vi "ReadTestList.vi"(10 "Model":string="7534-FE-FCT2") -> (1 "TestList":T1[](array[typedef]), 2 "size(s)":i32)   [LabVIEW 2013]
uses:
  TestVI/TestItemBox.ctl
  TestVI/TestItem.ctl
  Control/Buffer.vi
panel:
  out "Describe":string[](array[string])
  out "TestItem":string[](array[string])
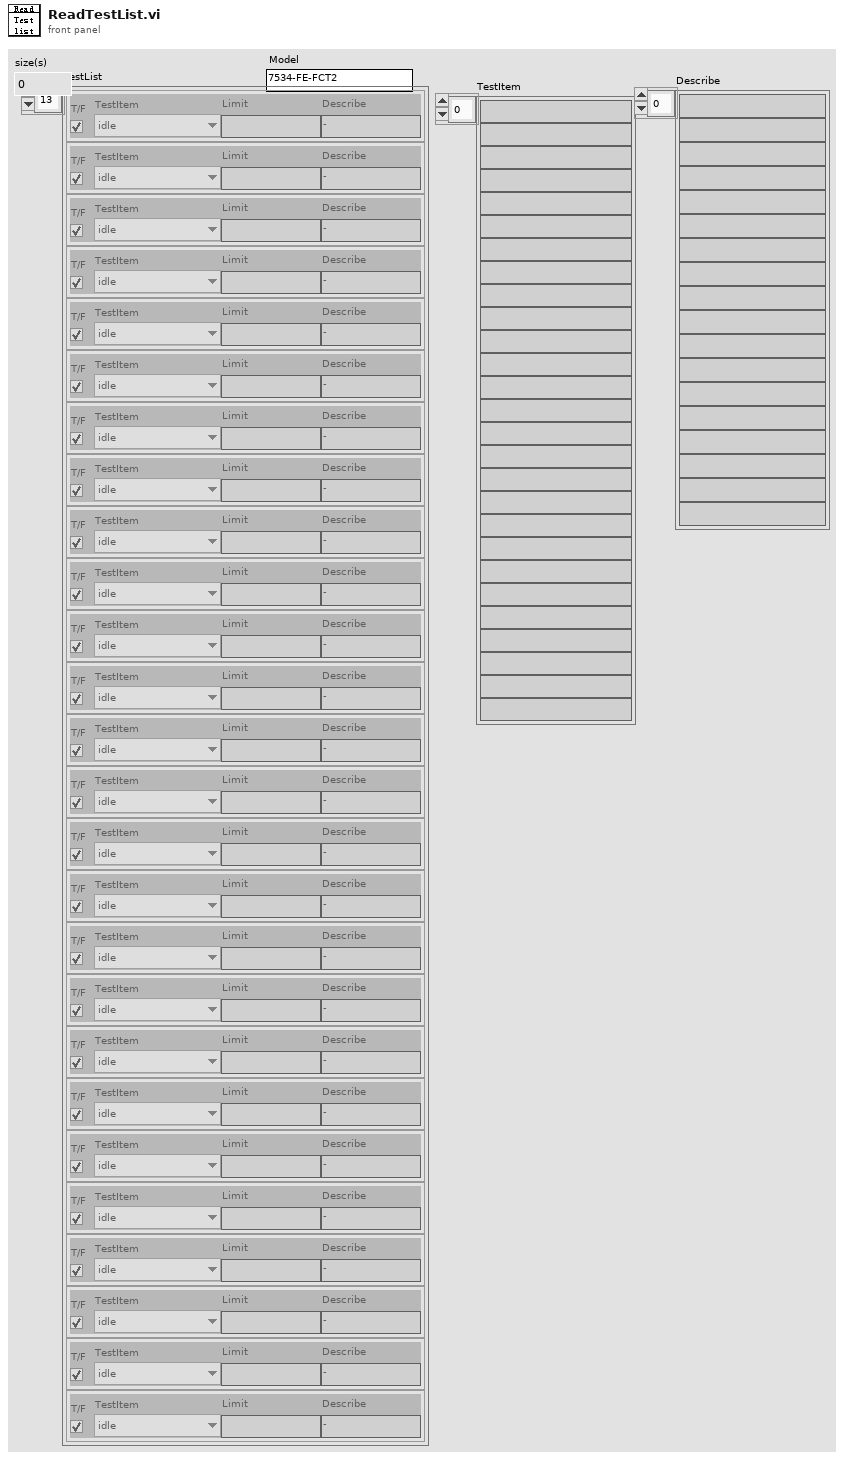
[diagram p1: front panel]
types:
  T1 = typedef "TestItemBox.ctl" = cluster{"T/F":bool, "TestItem":T2, "Limit":string, "Describe":string}
  T2 = typedef "TestItem.ctl" = enum16{"Dynamic_call", "idle", "Dialog", "Check_SF", "Delay", "Reset_HiPot", "HV_Test", "GB_Test", "Instrument_Write&Read_HIPOT", "Hipot_ReadResult", "Hipot_Close", "CheckModel", "ScanTestStart", "ScanMultChannel_DCV", "ScanOneChannel_DCV", "Diplay_TestList"}
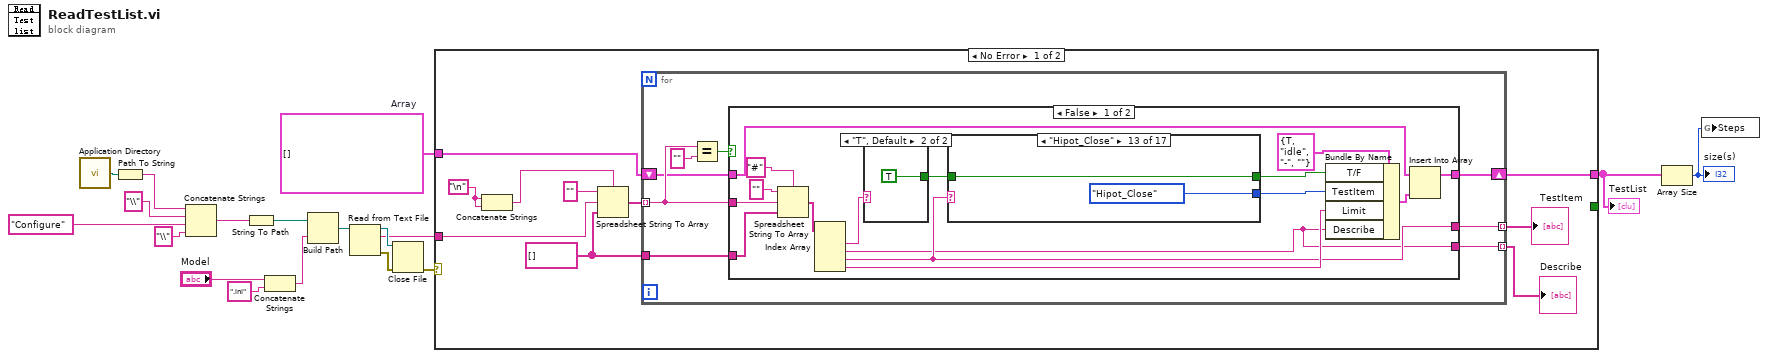
[diagram p0: block diagram]
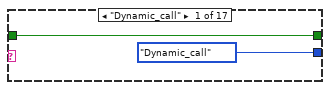
[diagram p2: hidden frame]
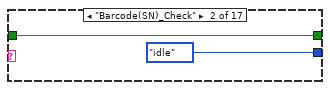
[diagram p3: hidden frame]
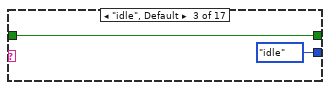
[diagram p4: hidden frame]
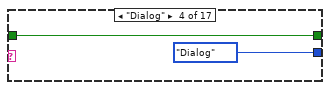
[diagram p5: hidden frame]
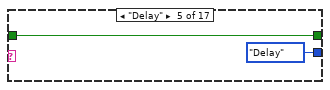
[diagram p6: hidden frame]
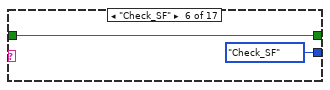
[diagram p7: hidden frame]
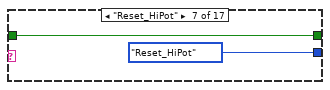
[diagram p8: hidden frame]
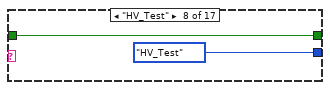
[diagram p9: hidden frame]
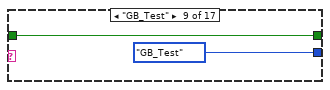
[diagram p10: hidden frame]
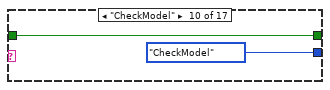
[diagram p11: hidden frame]
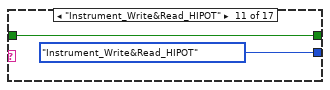
[diagram p12: hidden frame]
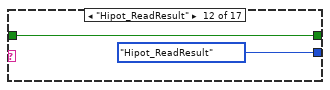
[diagram p13: hidden frame]
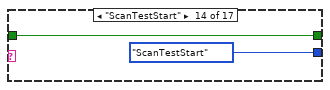
[diagram p14: hidden frame]
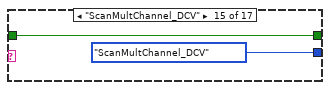
[diagram p15: hidden frame]
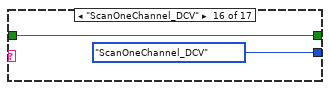
[diagram p16: hidden frame]
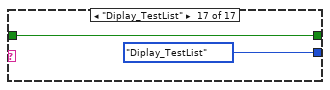
[diagram p17: hidden frame]
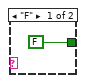
[diagram p18: hidden frame]
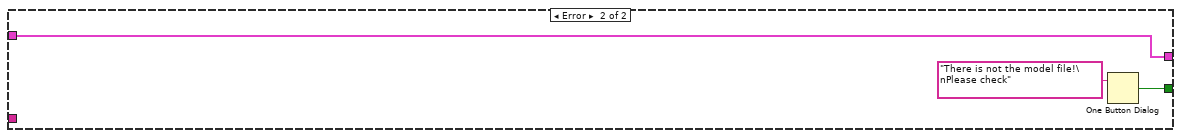
[diagram p20: hidden frame]
diagram:
  w2 = T1[] []  # Array
  n1 = call <vilib>:"Application Directory.vi"() -> ("Application Directory"=w15:path)
  n2 = Path To String(path=w15) -> (string=w14:string)
  n3 = Concatenate Strings(w14, "\\" ("string"), "Configure" ("string"), "\\" ("string")) -> (w11:string)
  n4 = String To Path(string=w11) -> (path=w10:path)
  n5 = Concatenate Strings("Model", ".ini" ("string")) -> (w7:string)
  n6 = Build Path(base path=w10, name or relative path=w7) -> (appended path=w1:path)
  n7 = Read from Text File(file (use dialog)=w1) -> (refnum out=w6:refnum<file>, text=w3:string, error out=w5:errorcluster)  [unwired: 3 in, 1 out]
  n8 = Close File(refnum=w6, error in=w5) -> (error out=w4:errorcluster)  [unwired: 1 out]
  n9 = case shown="No Error" w4 {
    tunnel: w3 -> [w28 _]
    tunnel: w2 -> [w24 w92]
    tunnel: [w23 w92] -> w17
    tunnel: [_ w90] -> _
    frame No Error {
      w22 = "\n"
      w25 = string[] []
      n10 = Concatenate Strings(w22, w22) -> (w21:string)
      n11 = Spreadsheet String To Array(delimiter (Tab)=w21, format string="", spreadsheet string=w28, array type (2D Dbl)=w25) -> (array=w26:string[])
      n12 = for {
        tunnel: w26 -> [w34] mode=indexing
        tunnel: w25 -> [w33]
        shift-right: [w31] -> w23
        shift-left: w24 -> [w32]
        tunnel: [w30] -> w20 mode=indexing
        tunnel: [w29] -> w19 mode=indexing
        n13 = Equal?(x=w34, y="") -> (x = y?=w35:bool)
        n14 = case shown="False" w35 {
          tunnel: w34 -> [w50 _]
          tunnel: w33 -> [w49 _]
          tunnel: w32 -> [w47 w89]
          tunnel: [w45 w89] -> w31
          tunnel: [w38 _] -> w30
          tunnel: [w37 _] -> w29
          frame False {
            n15 = Spreadsheet String To Array(delimiter (Tab)="#", format string="", spreadsheet string=w50, array type (2D Dbl)=w49) -> (array=w44:string[])
            n16 = Index Array(array=w44) -> (element #1=w43:string, element #2=w37:string, element #3=w38:string, element #4=w39:string)  [unwired: 4 in]
            n17 = case shown="\"T\", Default" w43 {
              tunnel: [FALSE TRUE] -> w41
              frame "F" {
              }
              frame "T", Default {
              }
            }
            n18 = case shown="\"Hipot_Close\"" w38 {
              tunnel: [w54 w56 w58 w60 w62 w64 w66 w68 w70 w72 w74 w76 w78 w80 w82 w84 w86] -> w42
              tunnel: w41 -> [w54 w56 w58 w60 w62 w64 w66 w68 w70 w72 w74 w76 w78 w80 w82 w84 w86]
              tunnel: [TestItem."Dynamic_call" ("TestItem") TestItem."idle" ("TestItem") TestItem."idle" ("TestItem") TestItem."Dialog" ("TestItem") TestItem."Delay" ("TestItem") TestItem."Check_SF" ("TestItem") TestItem."Reset_HiPot" ("TestItem") TestItem."HV_Test" ("TestItem") TestItem."GB_Test" ("TestItem") TestItem."CheckModel" ("TestItem") TestItem."Instrument_Write&Read_HIPOT" ("TestItem") TestItem."Hipot_ReadResult" ("TestItem") TestItem."Hipot_Close" ("TestItem") TestItem."ScanTestStart" ("TestItem") TestItem."ScanMultChannel_DCV" ("TestItem") TestItem."ScanOneChannel_DCV" ("TestItem") TestItem."Diplay_TestList" ("TestItem")] -> w40
              frame "Dynamic_call" {
              }
              frame "Barcode(SN)_Check" {
              }
              frame "idle", Default {
              }
              frame "Dialog" {
              }
              frame "Delay" {
              }
              frame "Check_SF" {
              }
              frame "Reset_HiPot" {
              }
              frame "HV_Test" {
              }
              frame "GB_Test" {
              }
              frame "CheckModel" {
              }
              frame "Instrument_Write&Read_HIPOT" {
              }
              frame "Hipot_ReadResult" {
              }
              frame "Hipot_Close" {
              }
              frame "ScanTestStart" {
              }
              frame "ScanMultChannel_DCV" {
              }
              frame "ScanOneChannel_DCV" {
              }
              frame "Diplay_TestList" {
              }
            }
            n19 = Bundle By Name(cluster=T1 {"T/F"=TRUE, "TestItem"=enum."idle", "Limit"="-", "Describe"=""} ("TestItemBox"), "T/F"=w42, "TestItem"=w40, "Limit"=w39, "Describe"=w37) -> (w46:T1)
            n20 = Insert Into Array(array=w47, new element=w46) -> (w45:T1[])  [unwired: 1 in]
          }
          frame True {
          }
        }
      }
      "TestItem" <- w20
      "Describe" <- w19
    }
    frame Error {
      n21 = One Button Dialog(message="There is not the model file!\nPlease check") -> (true=w90:bool)  [unwired: 1 in]
    }
  }
  "TestList" <- w17
  n22 = Array Size(array=w17) -> (size(s)=w18:i32)
  "size(s)" <- w18
  n23 = global write "Buffer.vi" "Steps"(w18) -> ()
